vi "Get Settings.vi"(8 "error in (no error)":errorcluster, 11 "DAQ_Engine in":refnum<class "DAQ_Engine.lvclass">) -> (0 "error out":errorcluster, 2 "Settings":T1={"Simulation"=FALSE, "Initial ErrReporting setting"=0, "Initial Measurement settings"={"Data Rate 9775"=3.0, "Data Rate 9215"=1200000.0, "Samples RMS 9215"=480000, "Samples RMS 9775"=3}, "Acquisition mode"=enum."3phase", "DemoMode"=FALSE, "RIO Device"=""} {"Initial ErrReporting setting" items=["DONTPRINT", "PRINTWARNINGS", "PRINTFATAL", "PRINTALL"]}, 3 "DAQ_Engine out":refnum<class "DAQ_Engine.lvclass">)   [LabVIEW 2019, in "DAQ_Engine.lvclass"]
doc: "Developed by Kevin Thompson\nkevin@thompsonengineering.net\n\nCopyright 2018\nThompson Engineering, LLC"
uses:
  DAQ_Engine.lvclass
  DataTypes/Settings--cluster.ctl
  Common/DataTypes/Measurement Config--cluster.ctl
  Common/DataTypes/Acquisition Mode--cluster.ctl
  DAQ_Engine.lvclass/DAQ_Engine.ctl
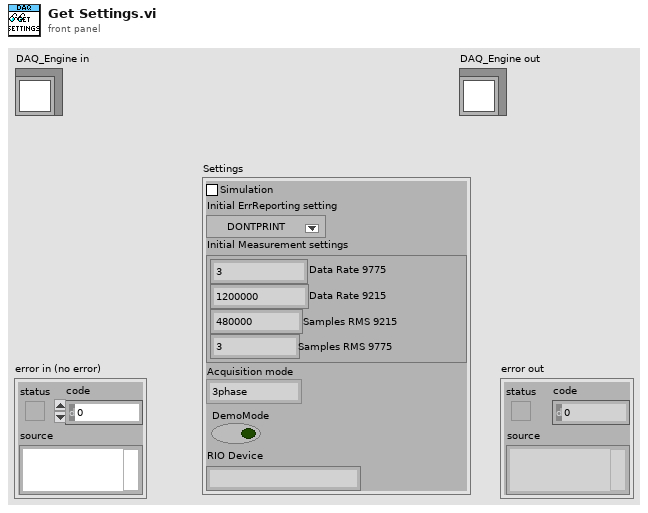
[diagram p1: front panel]
types:
  T1 = typedef "DAQ_Engine.lvclass/Settings--cluster.ctl" = cluster{"Simulation":bool, "Initial ErrReporting setting":i32, "Initial Measurement settings":T2, "Acquisition mode":T3, "DemoMode":bool, "RIO Device":string}
  T2 = typedef "Measurement Config--cluster.ctl" = cluster{"Data Rate 9775":dbl, "Data Rate 9215":dbl, "Samples RMS 9215":u32, "Samples RMS 9775":u32}
  T3 = typedef "Acquisition Mode--cluster.ctl" = enum16{"3phase", "Single"}
  T4 = typedef "DAQ_Engine.lvclass/ObjData--cluster.ctl" = cluster{"Settings":T1, "Public Events":T5, "Dependency":T6, "ReadData-placeholder":T7, "VISA-placeholder":refnum<visa-resource-name>, "MeasSettings":T2, "InverterDataAcqMode":T3, "RawDaqDataQ":T8, "Private Events":T9, "DAQState Data":T10}
  T5 = typedef "DAQ_Engine.lvclass/Public Events--cluster.ctl" = cluster{"DAQ_Engine.AsyncCmd Event":refnum<user-event>, "DAQ_Engine.AsyncMsg Event":refnum<user-event>, "stop process":refnum<user-event>, "DAQ_Engine.DAQStateChg Ev":refnum<user-event>, "DAQ_Engine.MeasSettingsChg Ev":refnum<user-event>, "DAQ_Engine.AcqModeChg Ev":refnum<user-event>}
  T6 = typedef "DAQ_Engine.lvclass/Dependency--cluster.ctl" = cluster{"Config":refnum<class "Config.lvclass">}
  T7 = typedef "DAQ_Engine.lvclass/Read Data--cluster.ctl" = cluster{"Data":dbl}
  T8 = typedef "RawDAQDataQRef--cluster.ctl" = refnum<queue>
  T9 = typedef "DAQ_Engine.lvclass/Private Events--cluster.ctl" = cluster{"PrivateAsync Ev":refnum<user-event>}
  T10 = typedef "DAQ_Engine.lvclass/DAQStateEvData--cluster.ctl" = cluster{"DAQState":T11, "vData":variant}
  T11 = typedef "DAQState--enum.ctl" = enum16{"Unknown", "Stopped", "Running", "Error"}
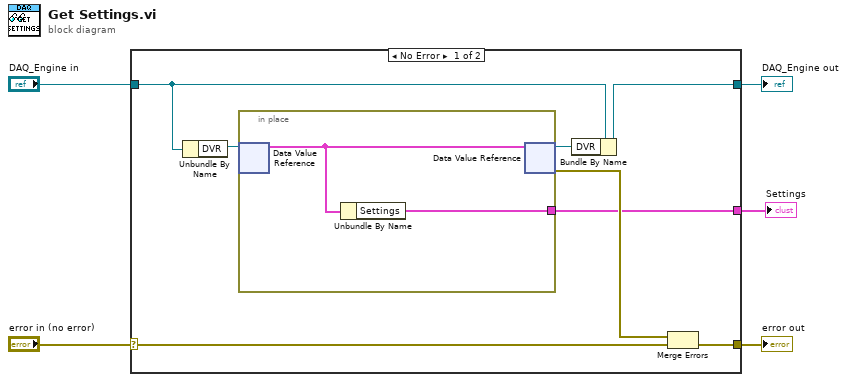
[diagram p0: block diagram]
diagram:
  n1 = case shown="No Error" "error in (no error)" {
    selector: "error in (no error)" -> [w13 w16]
    tunnel: [w8 w16] -> w4
    tunnel: [w9 w17] -> w2
    tunnel: "DAQ_Engine in" -> [w10 w17]
    tunnel: [w6 _] -> w1
    frame No Error {
      n2 = Unbundle By Name(w10) -> ("DVR"=w11:refnum<data-value>)
      n3 = in-place {
        in-place-border: [w14] -> w6
        n4 = in-place-dvr #1(w11) -> (w15:T4)  [unwired: 1 out]
        n5 = Unbundle By Name(w15) -> ("Settings"=w14:T1)
        n6 = in-place-dvr #1(w15) -> (w12:refnum<data-value>, w7:errorcluster)
      }
      n7 = Bundle By Name(cluster=w10, "DVR"=w12) -> (w9:refnum<class "DAQ_Engine.lvclass">)
      n8 = Merge Errors(w7, w13) -> (w8:errorcluster)
    }
    frame Error {
    }
  }
  "error out" <- w4
  "DAQ_Engine out" <- w2
  "Settings" <- w1
